vi "Send ADC.vi"(8 "error in (no error)":errorcluster, 9 "Channel":enum16{"2", "1"}(ring), 10 "VISA resource name":refnum<visa-resource-name>, 11 "Arduino in":refnum<class "Arduino.lvclass">) -> (0 "error out":errorcluster, 1 "Response":i32, 2 "VISA resource name 2":refnum<visa-resource-name>, 3 "Arduino out":refnum<class "Arduino.lvclass">)   [LabVIEW 2020, in "Arduino.lvclass"]
uses:
  Arduino.lvclass
  c99a2bd4-9158-49bc-add7-60c37fb6635b.vi
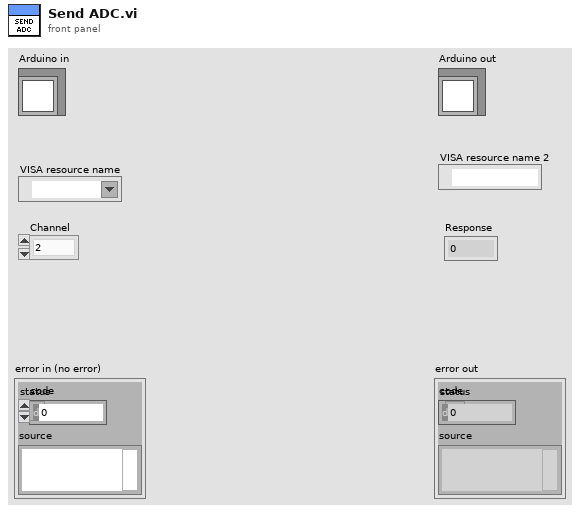
[diagram p1: front panel]
types:
  T1 = enum16{"Write", "Read", "Config", "Reset", "Close"}
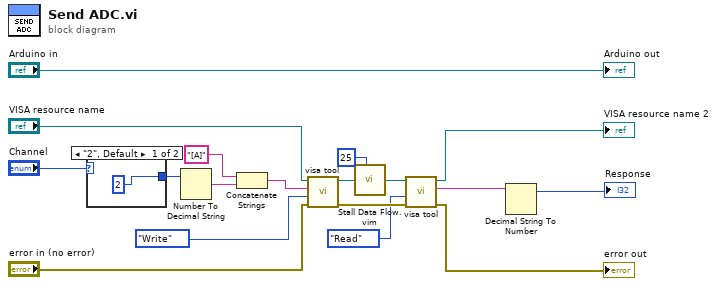
[diagram p0: block diagram]
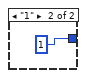
[diagram p2: hidden frame]
diagram:
  n1 = case shown="\"2\", Default" "Channel" {
    tunnel: [2 1] -> w1
    frame "2", Default {
    }
    frame "1" {
    }
  }
  n2 = Number To Decimal String(number=w1) -> (decimal integer string=w13:string)  [unwired: 1 in]
  n3 = Concatenate Strings("[A]" ("string"), w13) -> (w12:string)
  n4 = call "visa tool.vi"("error in (no error)"="error in (no error)", "Opciones"=T1."Write", "Write"=w12, "VISA com port"="VISA resource name") -> ("error out"=w6:errorcluster, "VISA com port 2"=w10:refnum<visa-resource-name>)  [unwired: 5 in, 1 out]
  n5 = call "Stall Data Flow.vim"("value in"=w10, "milliseconds to wait"=u32 25) -> ("value out"=w9:refnum<visa-resource-name>)  [unwired: 1 out]
  n6 = call "visa tool.vi"("error in (no error)"=w6, "Opciones"=T1."Read", "VISA com port"=w9) -> ("error out"=→"error out":errorcluster, "Read"=w5:string, "VISA com port 2"=→"VISA resource name 2":refnum<visa-resource-name>)  [unwired: 6 in]
  n7 = Decimal String To Number(string=w5) -> (offset past number=→"Response":i32)  [unwired: 2 in, 1 out]
  "Arduino out" <- "Arduino in"
